vi "Show User Interface.vi"(8 "error in (no error)":errorcluster, 9 "Process VI Refnums":refnum<vi>[](array[refnum]), 10 "Show UI":bool, 11 "SMO.UI.Example":refnum<class "SMO.UI.Example.lvclass">) -> (0 "error out":errorcluster, 3 "SMO.UI.Example out":refnum<class "SMO.UI.Example.lvclass">)   [LabVIEW 2013, in "SMO.UI.Example.lvclass"]
uses:
  SMO.UI.Example.lvclass
  SMO.UI.Example.lvclass/SMO.UI.Example.ctl
  src/SMO.UI/SMO.UI.lvclass
  src/SMO/SMO.lvclass
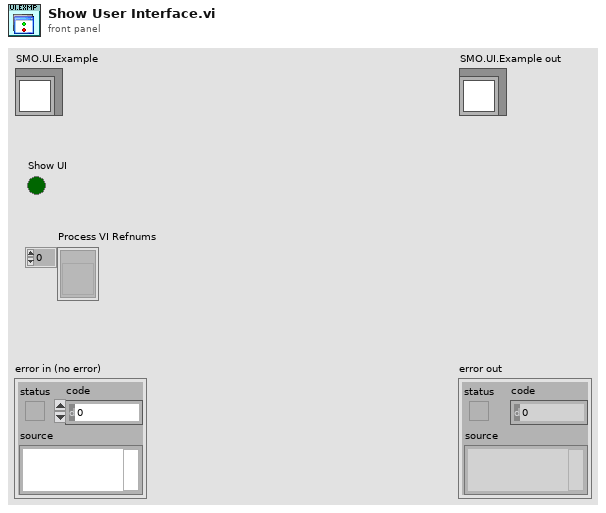
[diagram p1: front panel]
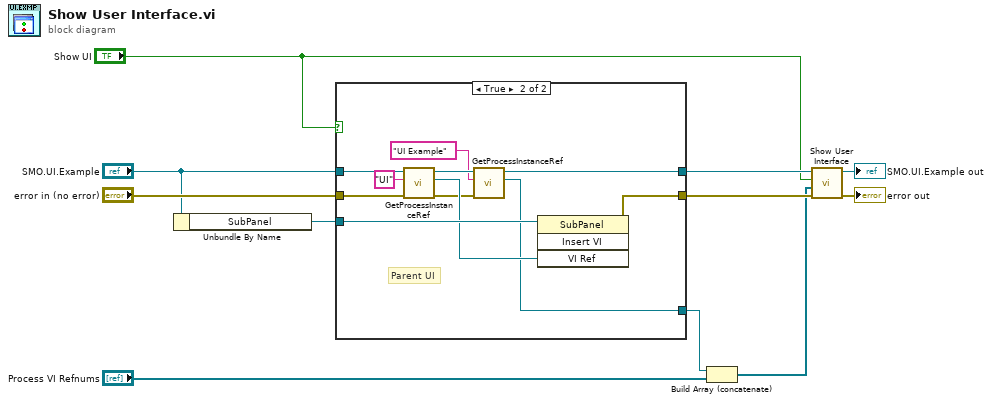
[diagram p0: block diagram]
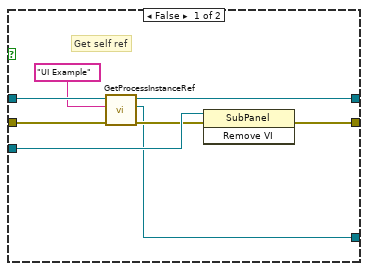
[diagram p2: hidden frame]
diagram:
  n1 = Unbundle By Name("SMO.UI.Example") -> ("SubPanel"=w2:refnum<vi>)
  n2 = case shown="True" "Show UI" {
    tunnel: "error in (no error)" -> [w17 w27]
    tunnel: [w13 w20] -> w8
    tunnel: "SMO.UI.Example" -> [w18 w28]
    tunnel: w2 -> [w19 w30]
    tunnel: [w12 w29] -> w6
    tunnel: [w15 w21] -> w1
    frame False {
      # "Get self ref"
      n3 = call "GetProcessInstanceRef.vi"("error in (no error)"=w17, "Process Name"="UI Example", "SMO"=w18) -> ("error out"=w16:errorcluster, "Process VI Refnum"=w15:refnum<vi>, "SMO out"=w13:refnum<class "SMO.UI.Example.lvclass">)  [unwired: 6 in]
      n4 = invoke on="Invoke Node" class="SubPanel" method="Remove VI"(reference=w19, error in=w16) -> (error out=w12:errorcluster)  [unwired: 1 in, 2 out]
    }
    frame True {
      # "Parent UI"
      n5 = call "GetProcessInstanceRef.vi"("error in (no error)"=w27, "Process Name"="UI", "SMO"=w28) -> ("error out"=w22:errorcluster, "Process VI Refnum"=w23:refnum<vi>, "SMO out"=w25:refnum<class "SMO.UI.Example.lvclass">)  [unwired: 6 in]
      n6 = call "GetProcessInstanceRef.vi"("error in (no error)"=w22, "Process Name"="UI Example", "SMO"=w25) -> ("Process VI Refnum"=w21:refnum<vi>, "SMO out"=w20:refnum<class "SMO.UI.Example.lvclass">)  [unwired: 6 in, 1 out]
      n7 = invoke on="Invoke Node" class="SubPanel" method="Insert VI"(reference=w30, "VI Ref"=w23) -> (error out=w29:errorcluster)  [unwired: 2 in, 3 out]
    }
  }
  n8 = Build Array (concatenate)(w1, "Process VI Refnums") -> (w4:refnum<vi>[])
  n9 = call-parent "Show User Interface.vi"("error in (no error)"=w6, "Process VI Refnums"=w4, "Show UI"="Show UI", "SMO.UI"=w8) -> ("error out"=→"error out":errorcluster, "SMO.UI out"=→"SMO.UI.Example out":refnum<class "SMO.UI.Example.lvclass">)  [unwired: 6 in]
